vi "Factory.vi"(8 "error in (no error)":errorcluster, 11 "Args":string[](array[string])) -> (0 "error out":errorcluster, 3 "Action":refnum<class "Action.lvclass">)   [LabVIEW 2018, in "neg-pkg.lvlib" / "Action.lvclass"]
uses:
  Action.lvclass
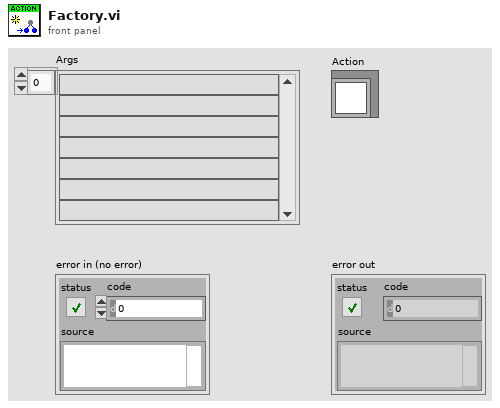
[diagram p1: front panel]
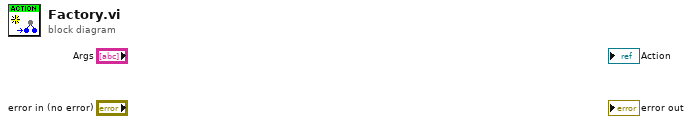
[diagram p0: block diagram]
diagram:
